vi "Get Event Name.vi"(11 "Event In":refnum<class "Event.lvclass">) -> (2 "Name":string, 3 "Event Out":refnum<class "Event.lvclass">)   [LabVIEW 2019, in "Event Source.lvlib" / "Event.lvclass"]
doc: "Get the name that defines the event.\n\n<b>IMPORTANT</b> - If no name is wired or the name string is empty, the name \"Generic\" will be used. This is to prevent errors with dictionary key name being empty."
uses:
  Event.lvclass
  Event.lvclass/Event.ctl
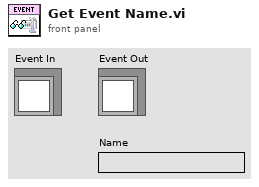
[diagram p1: front panel]
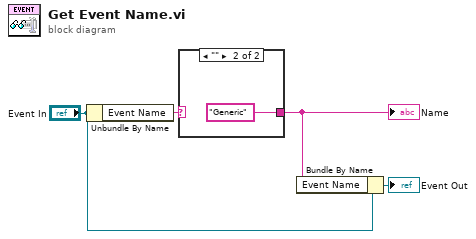
[diagram p0: block diagram]
diagram:
  n1 = Unbundle By Name("Event In") -> ("Event Name"=w4:string)
  n2 = case shown="\"\"" w4 {
    selector: w4 -> [w5 _]
    tunnel: [w5 "Generic"] -> w1
    frame Default {
    }
    frame "" {
    }
  }
  "Name" <- w1
  n3 = Bundle By Name(cluster="Event In", "Event Name"=w1) -> (→"Event Out":refnum<class "Event.lvclass">)
